vi "Get Setting.vi"(11 "PM_Group in":refnum<class "PM_Group.lvclass">) -> (2 "Setting PMG":T1 {"fililing voltage [V]" min=0.0 max=10.0 step=1.0; "fililing level %" min=0.0 max=10.0 step=1.0; "delta level" min=0.0 max=10.0 step=1.0; "Temp Close Water M21" min=0.0 max=200.0 step=1.0; "Temp Open Water M21" min=0.0 max=200.0 step=1.0; "Temp Turn OFF M24" min=0.0 max=200.0 step=1.0; "Temp Turn ON M24" min=0.0 max=200.0 step=1.0}, 3 "PM_Group out":refnum<class "PM_Group.lvclass">)   [LabVIEW 2019, in "PM_Group.lvclass"]
uses:
  PM_Group.lvclass
  TypeDef/GUI Setting PMG.ctl
  PM_Group.lvclass/PM_Group.ctl
panel:
  # "НС Охлаждения и отчистки (М24)"
  # "НС Подачи масла (М21)"
  # "НС Перекачки масла (М12)"
  # "Заправка"
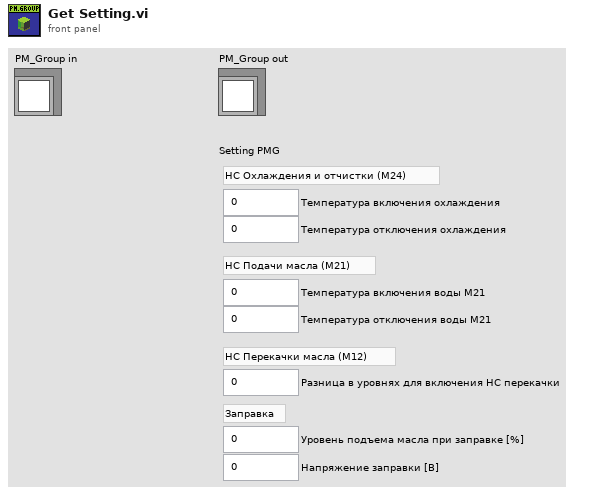
[diagram p1: front panel]
types:
  T1 = typedef "GUI Setting PMG.ctl" = cluster{"Temp Turn ON M24":dbl, "Temp Turn OFF M24":dbl, "Temp Open Water M21":dbl, "Temp Close Water M21":dbl, "delta level":dbl, "fililing level %":dbl, "fililing voltage [V]":dbl}
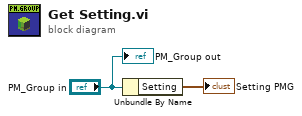
[diagram p0: block diagram]
diagram:
  n1 = Unbundle By Name("PM_Group in") -> ("Setting"=→"Setting PMG":T1)
  "PM_Group out" <- "PM_Group in"
